vi "Autonomous_Execution.vi"(0 "Queue Key":refnum<queue>, 5 "Autonomous_Queue":refnum<queue>, 11 "error in":errorcluster) -> (6 "Done":bool)   [LabVIEW 2020]
uses:
  Queue_Key_Data.ctl
  Robot_Subsystems.ctl
  Subsystems/Drive/Drive_Cluster.ctl
  Subsystems/Drive/Drive_Control_States.ctl
  Subsystems/Drive/Drive_Orientation_States.ctl
  Subsystems/Climber/Climber_Cluster.ctl
  Subsystems/Climber/Climber_Control_States.ctl
  Systems/Feeder/Feeder_Cluster.ctl
  Systems/Feeder/Feeder_Control_States.ctl
  Systems/Shooter/Determiner/Shooter_Cluster.ctl
  Systems/Shooter/Determiner/Shooter_Control_States.ctl
  Globals/Drive_Globals.vi
  Globals/Climber_Globals.vi
  Systems/Shooter/Determiner/Shooter_Globals.vi
  Globals/Feeder_Globals.vi
panel:
  in  "ignore previous (F)":bool
  in  "timeout in ms (-1)":i32=15
  out "notifiers out":refnum<notifier>[](array[refnum])
  # "AUTO:"
  # "AUTO:"
  # "AUTO STUFF:"
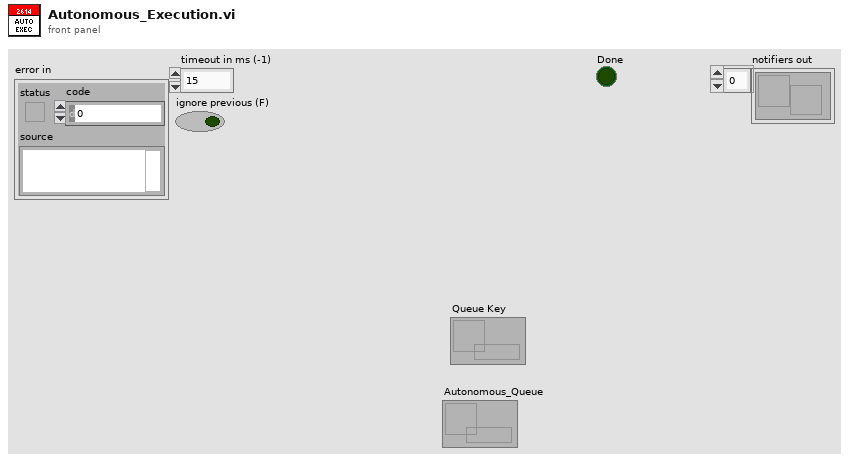
[diagram p1: front panel]
types:
  T1 = typedef "Queue_Key_Data.ctl" = cluster{"Operation Notifier":refnum<notifier>, "Subsystem":string, "Concurrent":bool}
  T2 = typedef "Robot_Subsystems.ctl" = cluster{"Drive_Cluster":T3, "Climber_Cluster":T6, "Feeder_Cluster":T8, "Shooter_Cluster":T10}
  T3 = typedef "Drive_Cluster.ctl" = cluster{"Control_State":T4, "Vertical_Throttle":dbl, "Lateral_Throttle":dbl, "Rotational_Throttle":dbl, "Strafe_In_Deadband":bool, "Rotation_In_Deadband":bool, "Orientation_State":T5, "Parameters":dbl[], "Step":i32, "Auto_Notifier":refnum<notifier>, "PathName":string}
  T4 = typedef "Drive_Control_States.ctl" = enum16{"No-Op", "Manual_Control", "Command_DriveDistanceAtAngle", "Command_DrivePath", "Command_SetRobotPose", "Command_Rotate"}
  T5 = typedef "Drive_Orientation_States.ctl" = enum16{"Robot-Oriented", "Field-Oriented"}
  T6 = typedef "Climber_Cluster.ctl" = cluster{"Control_State":T7, "Outer_Arm_Pivot_Throttle":dbl, "Outer_Arm_Elevator_Throttle":dbl, "Inner_Arm_Pivot_Throttle":dbl, "Enable_Climber_Sequence":bool, "Parameters":dbl[], "Auto_Notifier":refnum<notifier>, "Step":i32}
  T7 = typedef "Climber_Control_States.ctl" = enum16{"No-Op", "Manual_%Vbus", "Correct_Outer_Pivot_Offset", "Climbing_Sequence"}
  T8 = typedef "Feeder_Cluster.ctl" = cluster{"Firing":bool, "Load":bool, "Magazine_%Vbus":dbl, "Funnel_%Vbus":dbl, "Intake_%Vbus":dbl, "Manual_Extend":bool, "Outtake":bool, "Parameters":dbl[], "Auto_Notifier":refnum<notifier>, "Step":i32, "Control_States":T9}
  T9 = typedef "Feeder_Control_States.ctl" = enum16{"No-Op", "Manual", "Load", "Outtake", "Firing", "Test", "Command_Feed", "Command_Shoot"}
  T10 = typedef "Shooter_Cluster.ctl" = cluster{"Control_State":T11, "Shooting?":bool, "UpperGoal?":bool, "Limelight?":bool, "Flywheel_%Vbus":dbl, "Cowl_%Vbus":dbl, "Turret_%Vbus":dbl, "Parameters":dbl[], "Auto_Notifier":refnum<notifier>, "Step":i32, "Zero_Turret":bool}
  T11 = typedef "Shooter_Control_States.ctl" = enum16{"No-Op", "Limelight_Shooting", "Shoot_From_Pose", "Test", "Command_Shoot"}
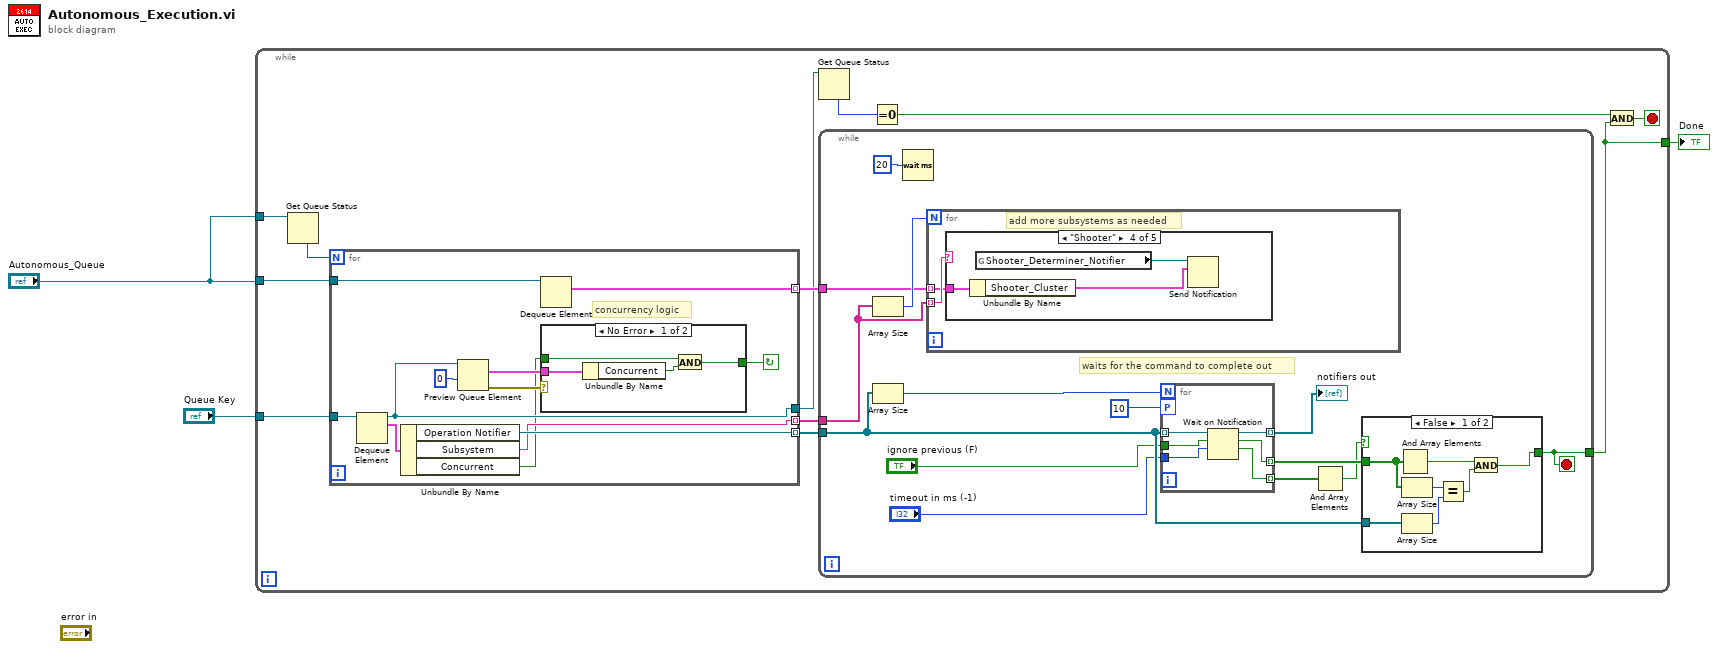
[diagram p0: block diagram]
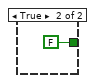
[diagram p2: hidden frame]
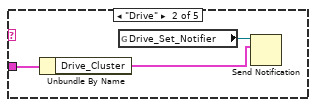
[diagram p4: hidden frame]
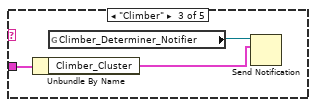
[diagram p5: hidden frame]
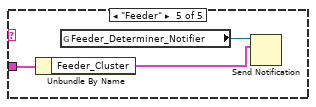
[diagram p6: hidden frame]
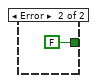
[diagram p7: hidden frame]
diagram:
  n1 = while {
    tunnel: "Queue Key" -> [w14]
    tunnel: "Autonomous_Queue" -> [w15]
    tunnel: "Autonomous_Queue" -> [w6]
    tunnel: [w4] -> w2
    stop <- w7 stop-if-true
    n2 = Get Queue Status(queue=w6) -> (# elements in queue=w9:i32)  [unwired: 2 in, 7 out]
    n3 = for {
      N: w9 -> [_]
      tunnel: w15 -> [w63]
      tunnel: w14 -> [w69]
      tunnel: [w60] -> w10 mode=indexing
      tunnel: [w64] -> w5
      tunnel: [w59] -> w12 mode=indexing
      tunnel: [w62] -> w11 mode=indexing
      stop <- w65 continue-if-true
      # "concurrency logic"
      n4 = Dequeue Element(queue=w69) -> (queue out=w64:refnum<queue>, element=w61:T1)  [unwired: 2 in, 2 out]
      n5 = Unbundle By Name(w61) -> ("Operation Notifier"=w60:refnum<notifier>, "Subsystem"=w59:string, "Concurrent"=w58:bool)
      n6 = Preview Queue Element(queue=w64, timeout in ms (-1)=0) -> (element=w68:T1, error out=w66:errorcluster)  [unwired: 1 in, 2 out]
      n7 = Dequeue Element(queue=w63) -> (element=w62:T2)  [unwired: 2 in, 3 out]
      n8 = case shown="No Error" w66 {
        tunnel: w68 -> [w71 _]
        tunnel: [w73 FALSE] -> w65
        tunnel: w58 -> [w72 _]
        frame No Error {
          n9 = Unbundle By Name(w71) -> ("Concurrent"=w70:bool)
          n10 = And(x=w72, y=w70) -> (x .and. y?=w73:bool)
        }
        frame Error {
        }
      }
    }
    n11 = Get Queue Status(queue=w5) -> (# elements in queue=w13:i32)  [unwired: 2 in, 7 out]
    n12 = while {
      tunnel: w12 -> [w24]
      tunnel: w11 -> [w23]
      tunnel: w10 -> [w25]
      tunnel: [w26] -> w4
      stop <- w26 stop-if-true
      # "waits for the command to complete out"
      n13 = Array Size(array=w24) -> (size(s)=w27:i32)
      n14 = Array Size(array=w25) -> (size(s)=w19:i32)
      n15 = Wait (ms)(milliseconds to wait=u32 20) -> ()  [unwired: 1 out]
      n16 = for {
        N: w27 -> [_]
        tunnel: w24 -> [w45] mode=indexing
        tunnel: w23 -> [w44] mode=indexing
        # "add more subsystems as needed"
        n17 = case shown="\"Shooter\"" w45 {
          tunnel: w44 -> [_ w48 w51 w54 w57]
          frame "No_Op", Default {
          }
          frame "Drive" {
            n18 = Unbundle By Name(w48) -> ("Drive_Cluster"=w47:T3)
            n19 = global read "Drive_Globals.vi" "Drive_Set_Notifier"() -> (w46:refnum<notifier>)
            n20 = Send Notification(notification=w47, notifier=w46) -> ()  [unwired: 1 in, 2 out]
          }
          frame "Climber" {
            n21 = Unbundle By Name(w51) -> ("Climber_Cluster"=w50:T6)
            n22 = global read "Climber_Globals.vi" "Climber_Determiner_Notifier"() -> (w49:refnum<notifier>)
            n23 = Send Notification(notification=w50, notifier=w49) -> ()  [unwired: 1 in, 2 out]
          }
          frame "Shooter" {
            n24 = Unbundle By Name(w54) -> ("Shooter_Cluster"=w53:T10)
            n25 = global read "Shooter_Globals.vi" "Shooter_Determiner_Notifier"() -> (w52:refnum<notifier>)
            n26 = Send Notification(notification=w53, notifier=w52) -> ()  [unwired: 1 in, 2 out]
          }
          frame "Feeder" {
            n27 = Unbundle By Name(w57) -> ("Feeder_Cluster"=w56:T8)
            n28 = global read "Feeder_Globals.vi" "Feeder_Determiner_Notifier"() -> (w55:refnum<notifier>)
            n29 = Send Notification(notification=w56, notifier=w55) -> ()  [unwired: 1 in, 2 out]
          }
        }
      }
      n30 = for {
        N: w19 -> [_]
        tunnel: w25 -> [w35] mode=indexing
        workers-P: 10 -> [_]
        tunnel: "timeout in ms (-1)" -> [w34]
        tunnel: "ignore previous (F)" -> [w33]
        tunnel: [w32] -> w22 mode=indexing
        tunnel: [w31] -> w29 mode=indexing
        tunnel: [w30] -> w17 mode=indexing
        n31 = Wait on Notification(notifier=w35, ignore previous (F)=w33, timeout in ms (-1)=w34) -> (notifier out=w32:refnum<notifier>, notification=w31:bool, timed out?=w30:bool)  [unwired: 1 in, 1 out]
      }
      "notifiers out" <- w22
      n32 = And Array Elements(Boolean array=w17) -> (logical AND=w28:bool)
      n33 = case shown="False" w28 {
        tunnel: [w41 FALSE] -> w26
        tunnel: w29 -> [w40 _]
        tunnel: w25 -> [w39 _]
        frame False {
          n34 = And Array Elements(Boolean array=w40) -> (logical AND=w42:bool)
          n35 = Array Size(array=w40) -> (size(s)=w38:i32)
          n36 = Array Size(array=w39) -> (size(s)=w37:i32)
          n37 = Equal?(x=w38, y=w37) -> (x = y?=w36:bool)
          n38 = And(x=w42, y=w36) -> (x .and. y?=w41:bool)
        }
        frame True {
        }
      }
    }
    n39 = Equal To 0?(x=w13) -> (x = 0?=w8:bool)
    n40 = And(x=w8, y=w4) -> (x .and. y?=w7:bool)
  }
  "Done" <- w2
